vi "action.vi"(0 "MoAgSy_Visitor_stop":refnum<class "MoAgSy_Visitor_stop.lvclass">, 2 "HGF_Visitable":refnum<class "HGF_Visitable.lvclass">, 5 "error in (no error)":errorcluster) -> (14 "dup MoAgSy_Visitor_stop":refnum<class "MoAgSy_Visitor_stop.lvclass">, 16 "dup HGF_Visitable":refnum<class "HGF_Visitable.lvclass">, 19 "error out":errorcluster)   [LabVIEW 2009, in "MoAgSy.lvlib" / "MoAgSy_Visitor_stop.lvclass"]
doc: "This is a dynamic dispatch VI that is called from Visitor.visit(). It will call member VIs of Visitable to perform the requested action which means: calling public methods of Visitable child class.\n\n<B>Hint:</B> This method is abstract and need to be implemented by child classes."
uses:
  MoAgSy_Visitor_stop.lvclass
  HGF_BaseClasses/HGF_Visitable/HGF_Visitable.lvclass
  MoAgSy_AgentBase/MoAgSy_AgentBase.lvclass
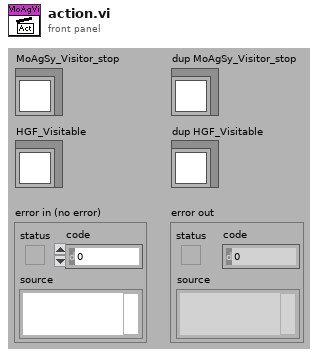
[diagram p1: front panel]
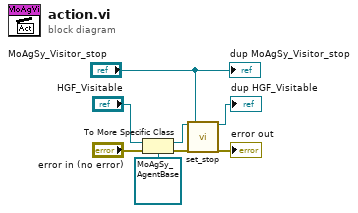
[diagram p0: block diagram]
diagram:
  n1 = To More Specific Class(target class=refnum<class "MoAgSy_AgentBase.lvclass"> refnum ("HGF_AgentBaseClasses.lvlib:HGF_Agent.lvclass"), reference="HGF_Visitable", error in="error in (no error)") -> (specific class reference=w5:refnum<class "MoAgSy_AgentBase.lvclass">, error out=w3:errorcluster)
  n2 = call "set_stop.vi"("HGF_Agent.lvclass in"=w5, "error in (no error)"=w3, "MoAgSy_Visitor_stop in"="MoAgSy_Visitor_stop") -> ("HGF_Agent.lvclass out"=→"dup HGF_Visitable":refnum<class "MoAgSy_AgentBase.lvclass">, "error out"=→"error out":errorcluster)  [unwired: 1 in, 14 out]
  "dup MoAgSy_Visitor_stop" <- "MoAgSy_Visitor_stop"
